vi "Filtro_EMA_(SubVI).vi"(11 "Entrada":dbl) -> (3 "Salida":dbl)   [LabVIEW 2020]
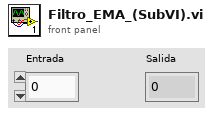
[diagram p1: front panel]
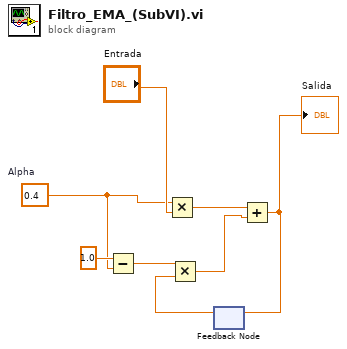
[diagram p0: block diagram]
diagram:
  w1 = 0.4  # Alpha
  n1 = Subtract(x=1.0, y=w1) -> (x-y=w5:dbl)
  n2 = Multiply(x=w1, y="Entrada") -> (x*y=w3:dbl)
  n3 = feedback #1() -> (w6:dbl)  [unwired: 1 in]
  n4 = Multiply(x=w5, y=w6) -> (x*y=w2:dbl)
  n5 = Add(x=w3, y=w2) -> (x+y=w7:dbl)
  "Salida" <- w7
  n6 = feedback-in #1(w7) -> ()
